vi "Disconnect.vi"(8 "error in (no error)":errorcluster, 11 "Stepper3D in":refnum<class "Stepper3D.lvclass">) -> (0 "error out":errorcluster, 3 "Stepper3D out":refnum<class "Stepper3D.lvclass">)   [LabVIEW 2014, in "Stepper3D.lvclass"]
uses:
  Stepper3D.lvclass
  Stepper3D.lvclass/Stepper3D.ctl
  Libs/stepper3D.lib/stepper3D.lvlib
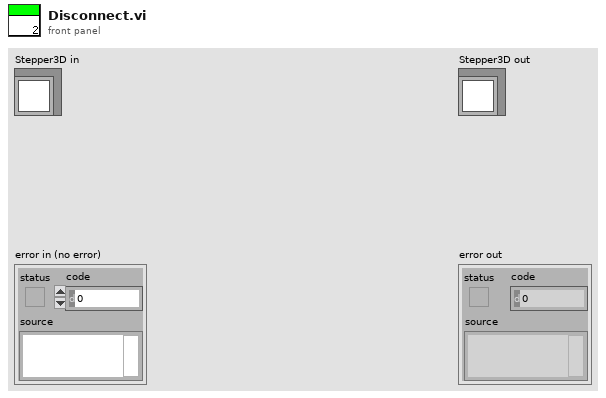
[diagram p1: front panel]
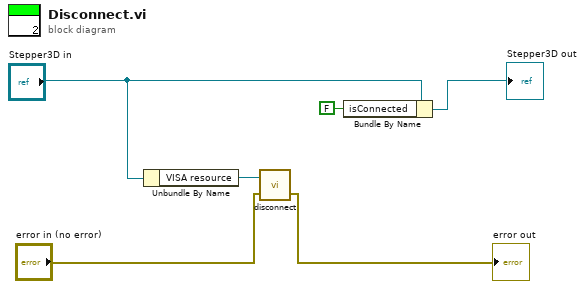
[diagram p0: block diagram]
diagram:
  n1 = Unbundle By Name("Stepper3D in") -> ("VISA resource"=w6:refnum<visa-resource-name>)
  n2 = call "disconnect.vi"("error in"="error in (no error)", "VISA resource name"=w6) -> ("error out"=→"error out":errorcluster)  [unwired: 1 in]
  n3 = Bundle By Name(cluster="Stepper3D in", "isConnected"=FALSE) -> (→"Stepper3D out":refnum<class "Stepper3D.lvclass">)
